vi "CollisionAvoidanceEnabled_set.vi"(8 "error in (no error)":errorcluster, 10 "Enabled? (T)":bool=TRUE) -> (0 "error out":errorcluster)   [LabVIEW 2009, in "Main.lvlib" / "MainVariables.lvlib"]
uses:
  OWNCAN/MainVariables.lvlib
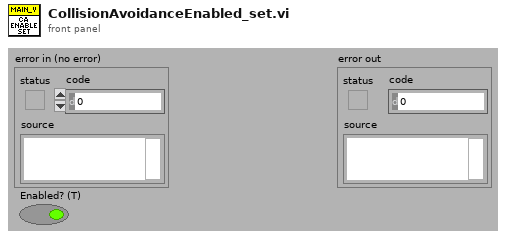
[diagram p1: front panel]
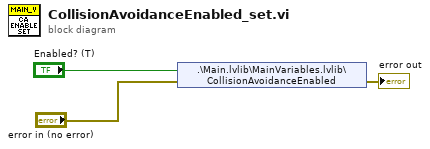
[diagram p0: block diagram]
diagram:
  n1 = shared-variable ".\\Main.lvlib\\MainVariables.lvlib\\CollisionAvoidanceEnabled"("Enabled? (T)", error in="error in (no error)") -> (error out=→"error out":errorcluster)
